vi "SCLN_MessageToServer.vi"(2 "error in (no error)":errorcluster, 3 "Message":string, 4 "Server Name":string) -> (0 "error out":errorcluster, 1 "Index for Response":i32)   [LabVIEW 2015]
uses:
  SCLN_RW_Select.ctl
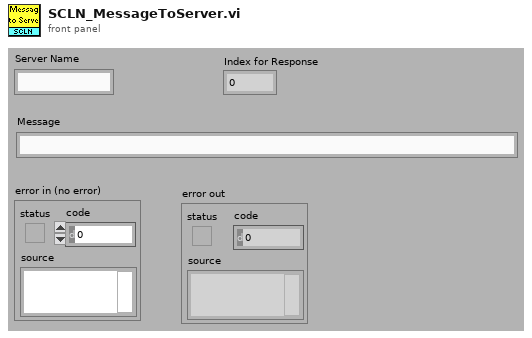
[diagram p1: front panel]
types:
  T1 = typedef "SCLN_RW_Select.ctl" = enum16{"Read", "Write"}
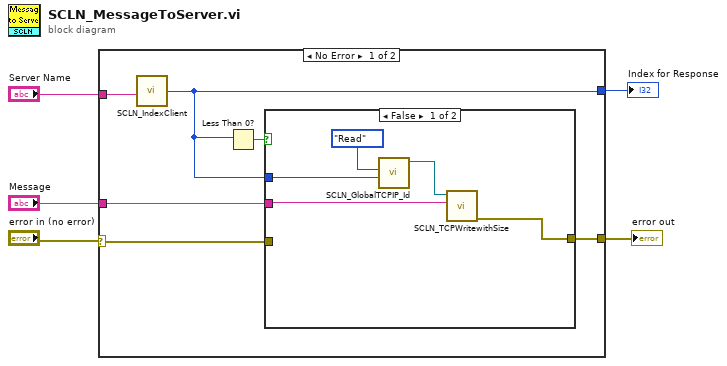
[diagram p0: block diagram]
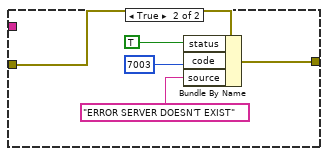
[diagram p2: hidden frame]
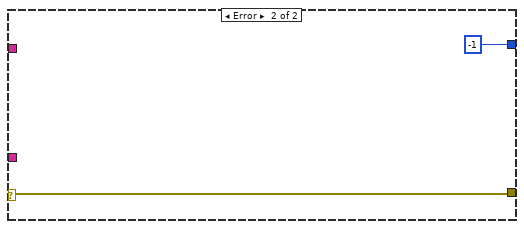
[diagram p3: hidden frame]
diagram:
  n1 = case shown="No Error" "error in (no error)" {
    selector: "error in (no error)" -> [w6 w22]
    tunnel: [w8 -1] -> w5
    tunnel: "Server Name" -> [w11 _]
    tunnel: [w9 w22] -> w2
    tunnel: "Message" -> [w7 _]
    frame No Error {
      n2 = call "SCLN_IndexClient.vi"("Server Name"=w11) -> ("Index"=w8:i32)
      n3 = Less Than 0?(x=w8) -> (x < 0?=w10:bool)
      n4 = case shown="False" w10 {
        tunnel: [w12 w18] -> w9
        tunnel: w8 -> [w15 _]
        tunnel: w7 -> [w13 _]
        tunnel: w6 -> [_ w17]
        frame False {
          n5 = call "SCLN_GlobalTCPIP_Id.vi"("Element"=w15, "Operation"=SCLN_RW_Select."Read" ("GBL_RW")) -> ("TCPIP_Id Read"=w14:refnum<k5>)  [unwired: 2 in, 1 out]
          n6 = call "SCLN_TCPWritewithSize.vi"("data in"=w13, "connection ID"=w14) -> ("error out"=w12:errorcluster)  [unwired: 7 in, 2 out]
        }
        frame True {
          n7 = Bundle By Name(cluster=w17, "status"=TRUE, "code"=7003, "source"="ERROR SERVER DOESN'T EXIST") -> (w18:errorcluster)
        }
      }
    }
    frame Error {
    }
  }
  "Index for Response" <- w5
  "error out" <- w2
